vi "QuP Multiplexer Control.vi"(11 "Do full quit? (T)":bool=TRUE) -> ()   [LabVIEW 2020, in "QuPMXdriver.lvlib"]
uses:
  QuPMXdriver.lvlib
  91754cce-ab52-4237-b78a-64c01c446f44.vi
  32ad12f4-2c8c-4504-800a-0d774754ae80.vi
  bf4f7028-8ca7-4759-aadb-7144e2be3c91.vi
  040f1b57-66c1-4072-aa26-6ea72dd8171f.vi
  6aed5eb3-691d-4dc6-b830-00691c629857.vi
  Sequence Editor.vi
  <vilib>/Comparison/Equal/Equal Functor/Equal Functor.lvclass
panel:
  in  "disconnect":bool
  out "dummy for event \"check channels\"":bool
  in  "Set to sequence line:":i32=2 min=1 step=1
  in  "set sq line":bool
  out "Connected\nboards":bool[](array[boolean])
  in  "Get sq from MX":bool
  in  "Load sq to MX":bool
  in  "no sequences get":bool
  out "Number of sequence lines:":i32 min=0 step=1
  in  "sequence editor":bool
  out "Guards ref array":refnum<vi>[][](array[refnum])
  in  "G5C1":bool
  in  "G5C2":bool
  in  "G6C1":bool
  in  "G6C2":bool
  in  "G4C1":bool
  in  "G4C2":bool
  in  "G3C1":bool
  in  "G3C2":bool
  in  "G2C1":bool
  in  "G2C2":bool
  in  "G1C1":bool
  in  "G1C2":bool
  out "No. of connected slave boards:":u32
  out "Slaves ref array":refnum<vi>[][](array[refnum])
  in  "S5C1":bool
  in  "S5C2":bool
  in  "S6C1":bool
  in  "S6C2":bool
  in  "S4C1":bool
  in  "S4C2":bool
  in  "S3C1":bool
  in  "S3C2":bool
  in  "S2C1":bool
  in  "S2C2":bool
  in  "S1C1":bool
  in  "S1C2":bool
  in  "connect":bool
  in  "Get Status":bool
  out "Ready?":bool=TRUE
  out "Enabled":bool=TRUE
  in  "check channels":bool
  in  "delay get":bool
  in  "delay set":bool
  in  "Enable\nDelay (ms)":dbl=2.0 min=0.8
  in  "timer get":bool
  in  "timer set":bool
  in  "Timer (ms)":i32=1000 min=0 step=1
  in  "Trigger polarity":enum32{"Positive", "Negative"}(radio)
  in  "Trigger source":enum32{"Internal", "External"}(radio)
  out "FP":refnum<vi>[](array[refnum])
  in  "Operation":enum32{"Remote", "Local"}(radio)=enum."Local"
  out "ID":string
  in  "reset":bool
  in  "clear":bool
  in  "stop":bool
  in  "start":bool
  in  "resume":bool
  in  "pause":bool
  in  "Close":bool
  out "error":errorcluster
  in  "VISA":refnum<visa-resource-name>
  # "Channels"
  # "Properties"
  # "Slave boards"
  # "1       2      3      4      5      6"
  # "Channel 1"
  # "Channel 2"
  # "1       2      3      4      5      6"
  # "Guards"
  # "Channel 1"
  # "These are buttons,\nclick it!"
  # "Channel 2"
  # "Sequence"
  # "Error"
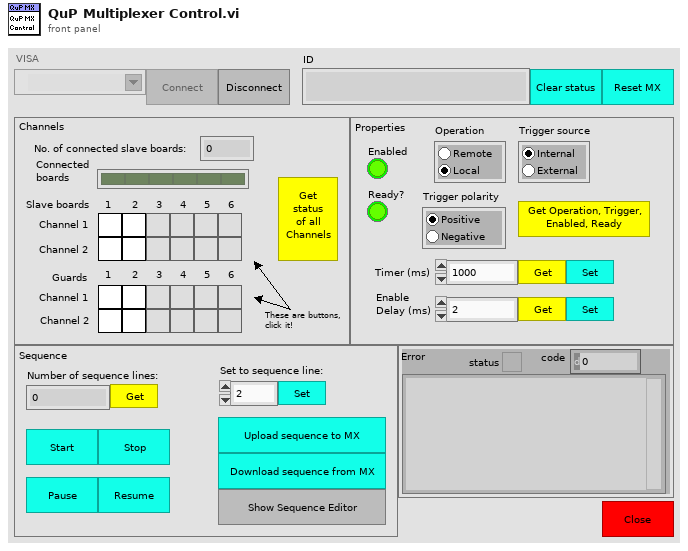
[diagram p1: front panel]
types:
  T1 = enum8{"Enabled", "Disabled", "Disabled and Grayed Out"}
  T2 = enum32{"Invalid", "Standard", "Closed", "Hidden", "Minimized", "Maximized"}
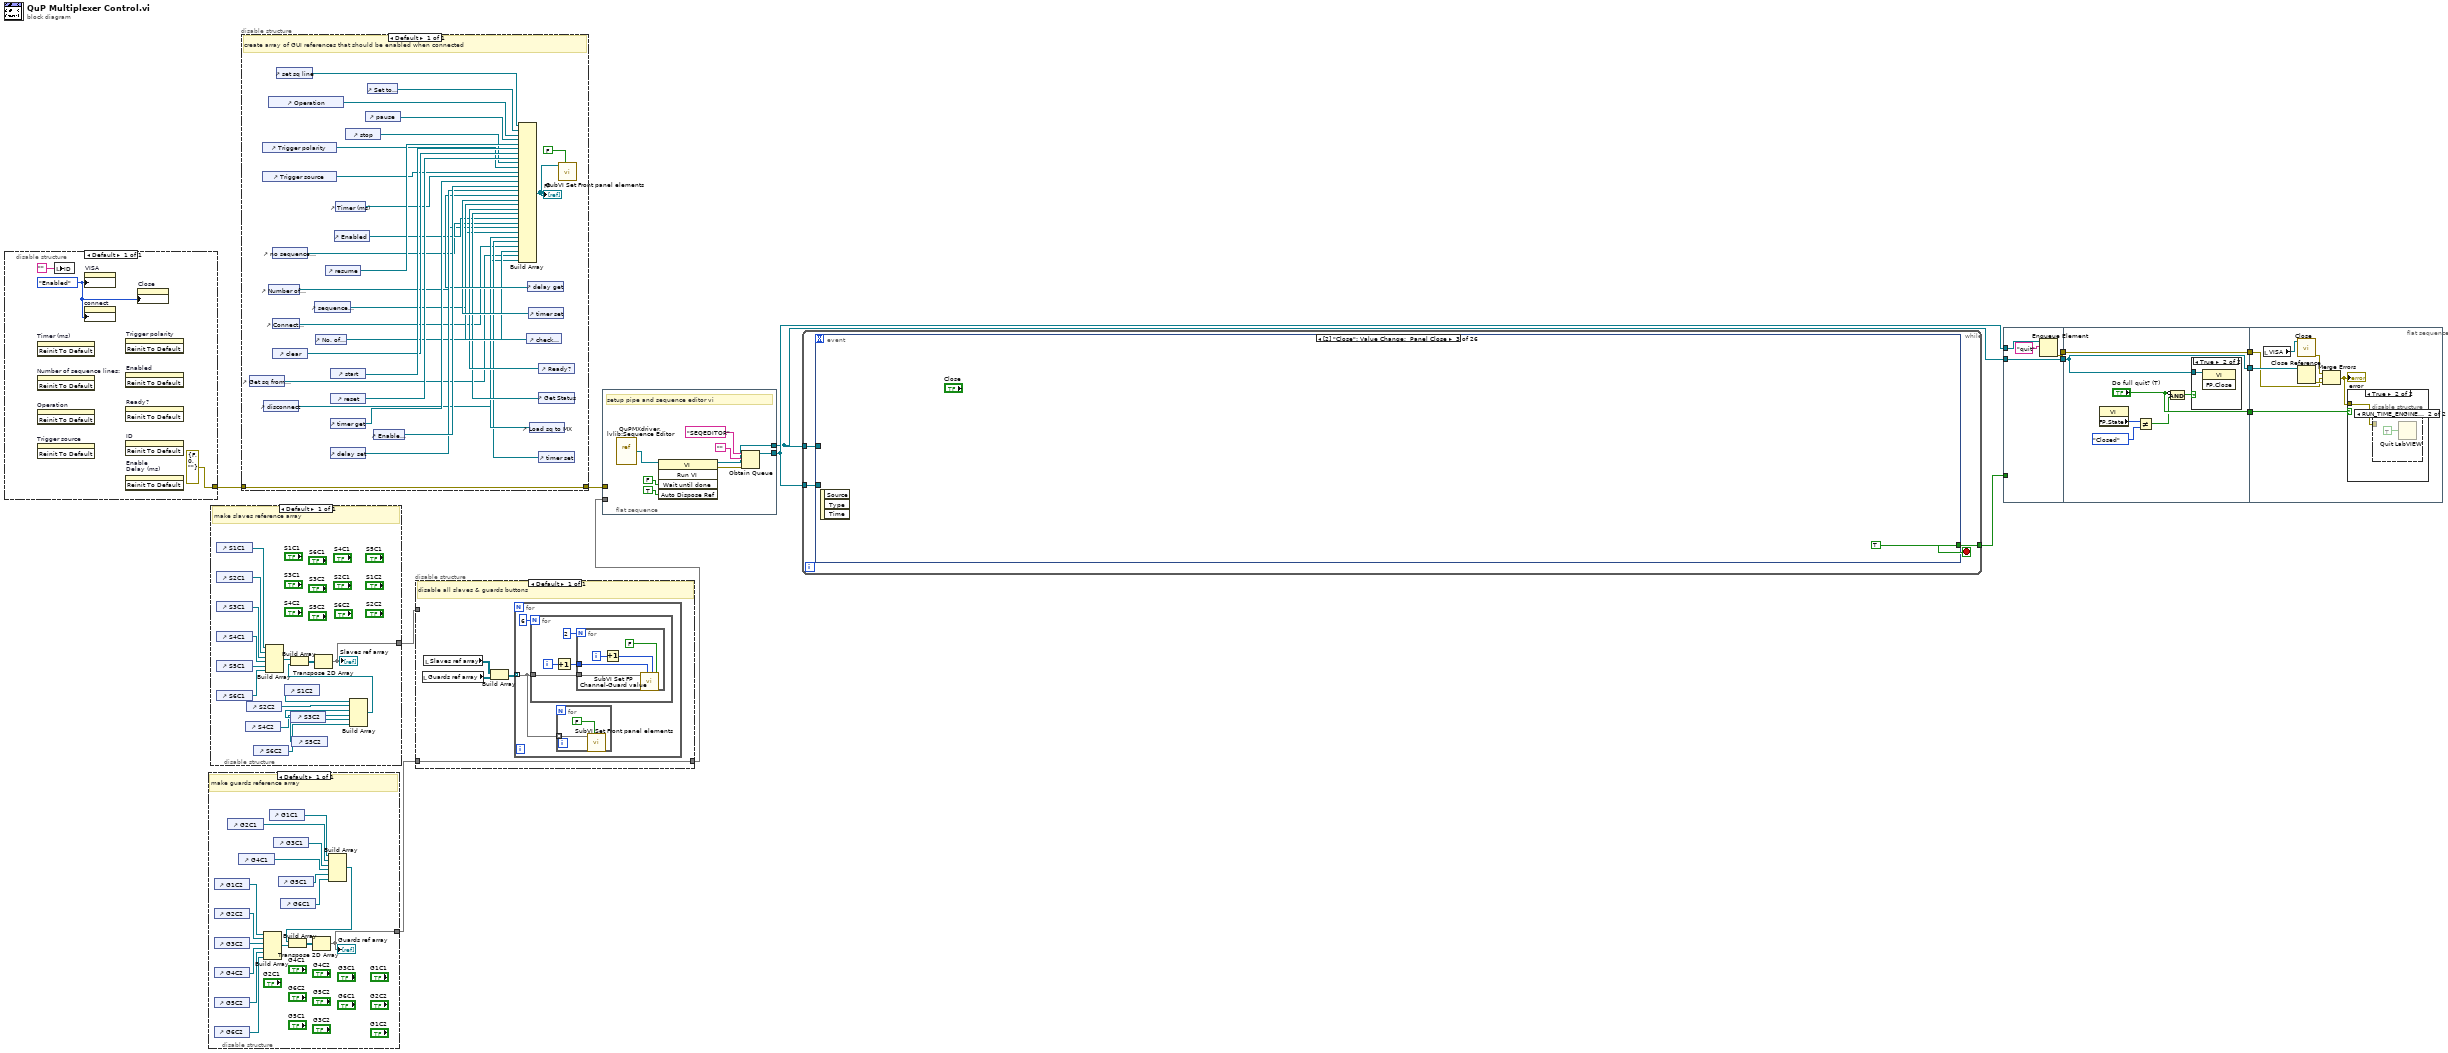
[diagram p0: block diagram]
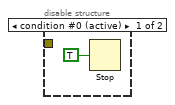
[diagram p4: hidden frame]
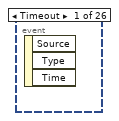
[diagram p5: hidden frame]
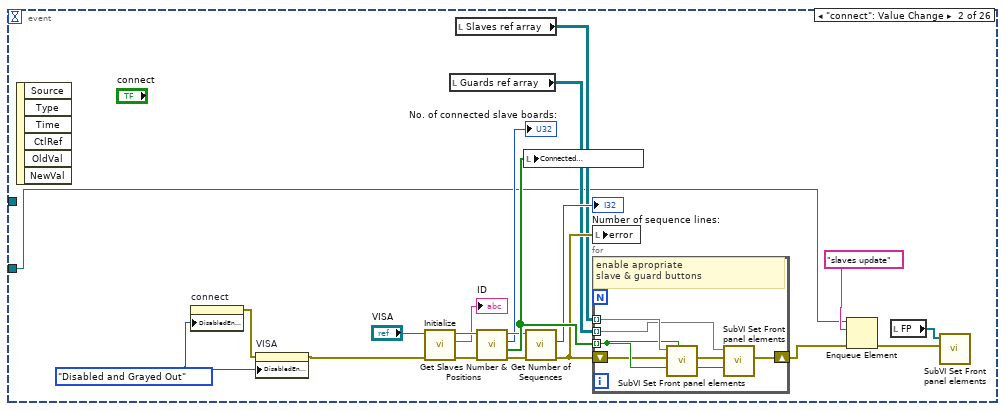
[diagram p6: hidden frame]
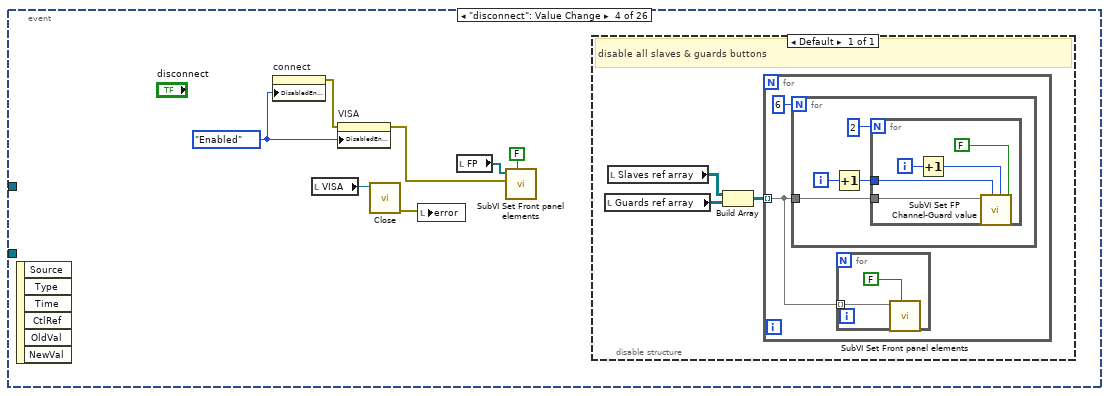
[diagram p7: hidden frame]
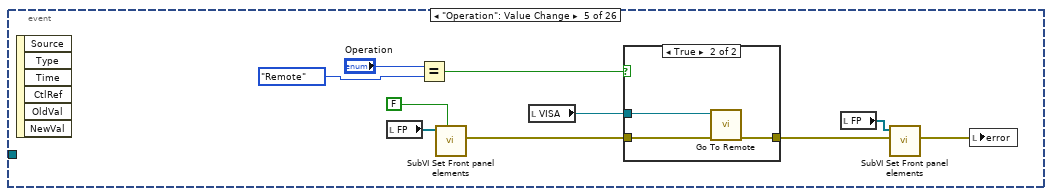
[diagram p8: hidden frame]
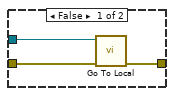
[diagram p9: hidden frame]
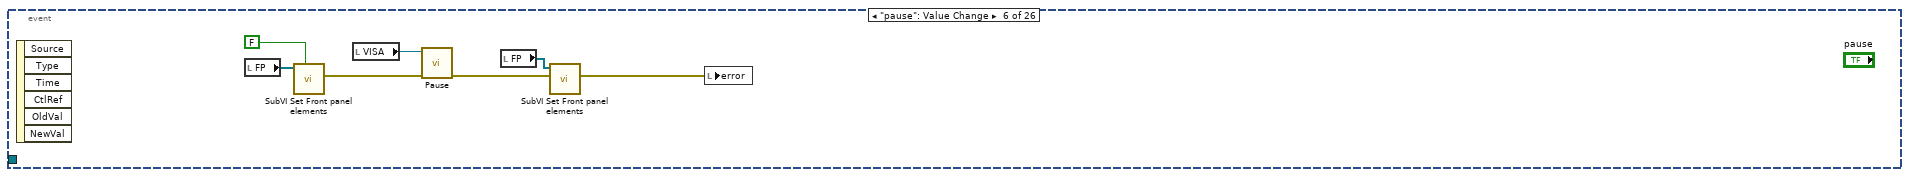
[diagram p10: hidden frame]
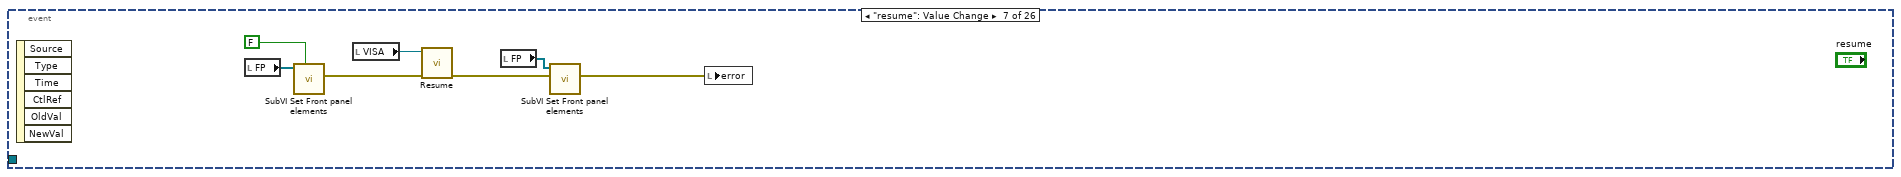
[diagram p11: hidden frame]
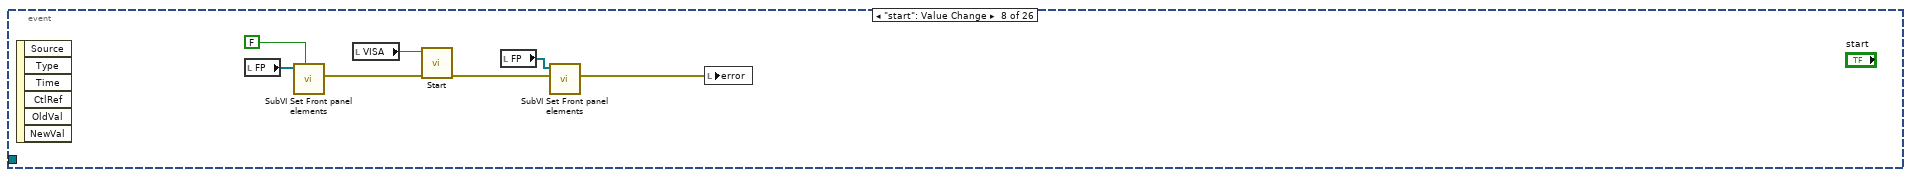
[diagram p12: hidden frame]
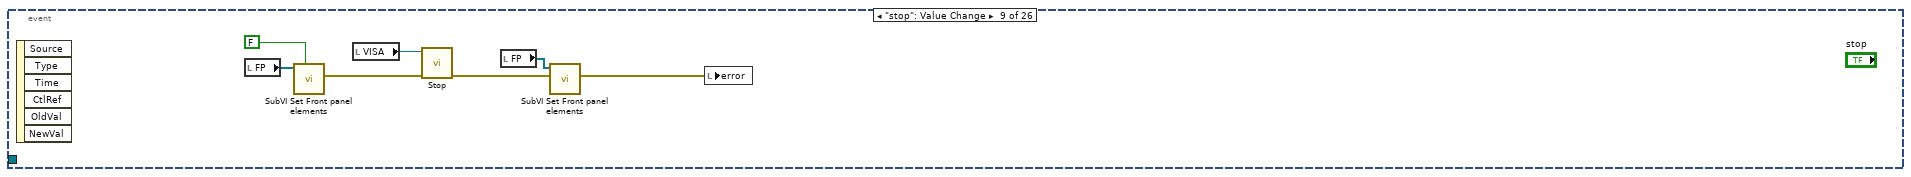
[diagram p13: hidden frame]
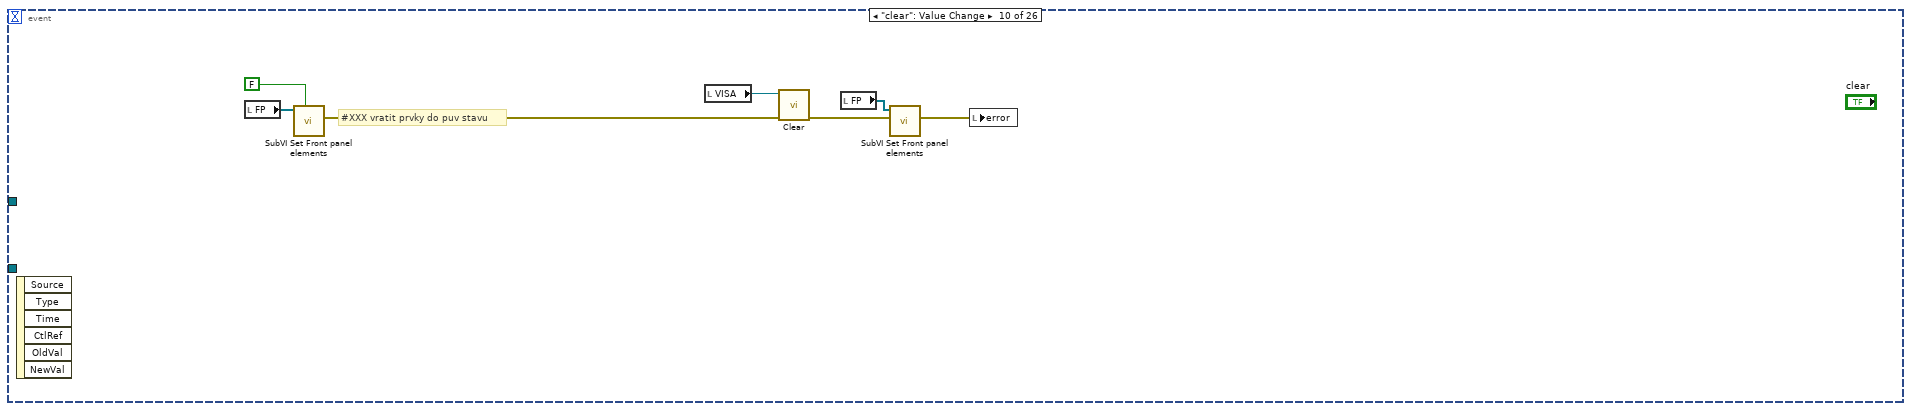
[diagram p14: hidden frame]
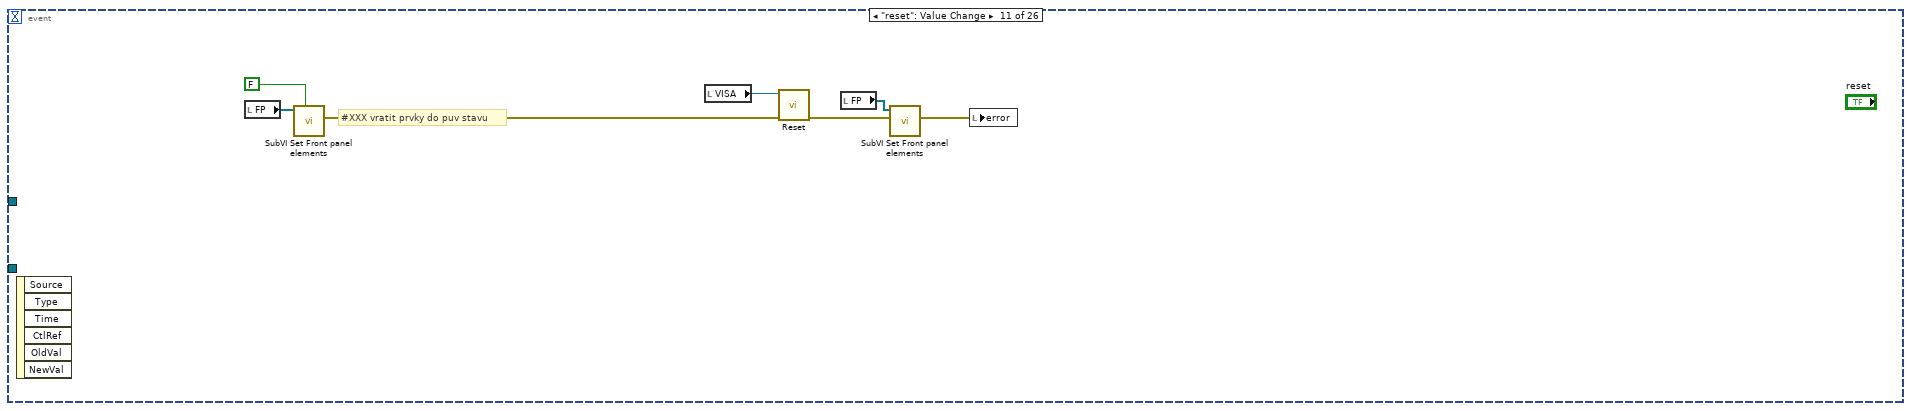
[diagram p15: hidden frame]
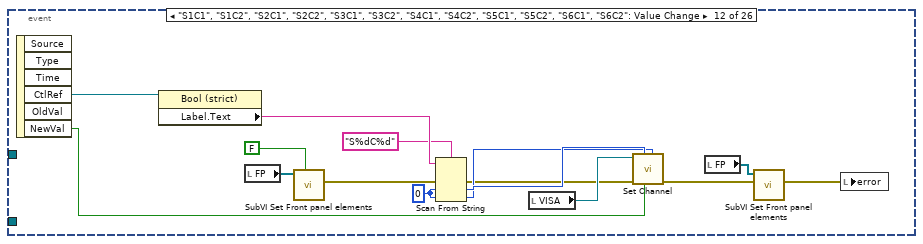
[diagram p16: hidden frame]
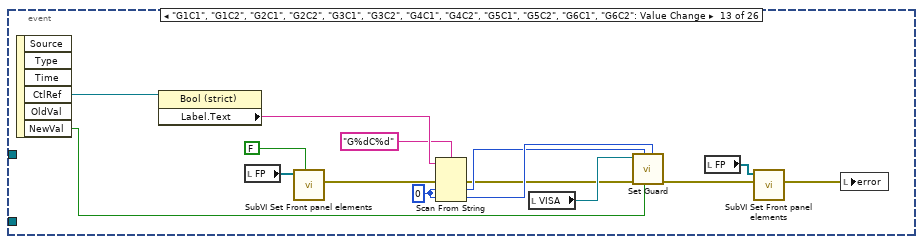
[diagram p17: hidden frame]
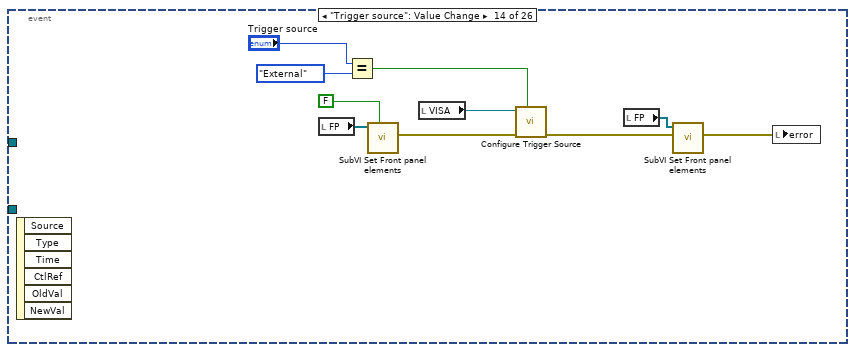
[diagram p18: hidden frame]
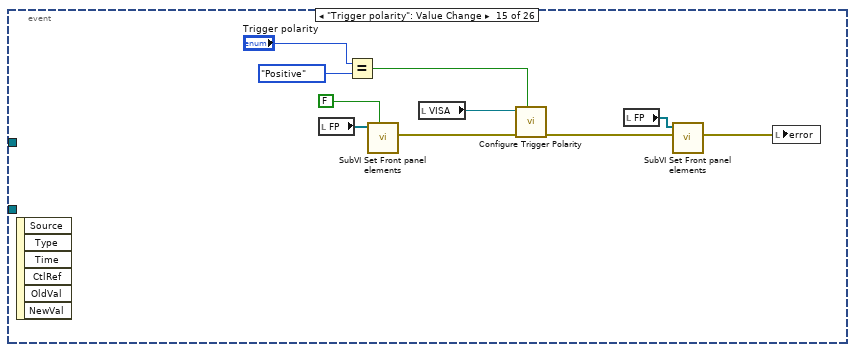
[diagram p19: hidden frame]
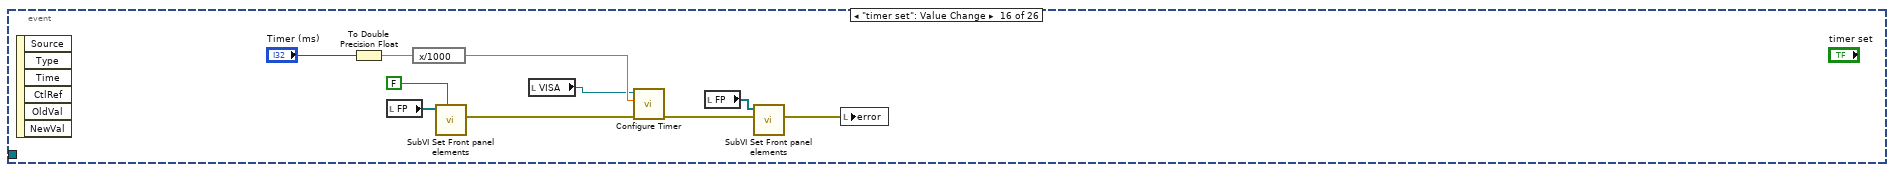
[diagram p20: hidden frame]
diagram:
  n1 = disable-structure shown="Default" {
    disable-tunnel: [errorcluster {"status"=FALSE, "code"=0, "source"=""} ("error in (no error)")] -> w8
    frame Enabled {
      w14 = T1."Enabled" ("Disabled")
      n2 = invoke on="Timer (ms)" class="DigNum (strict)" method="Reinit To Default"() -> ()  [unwired: 3 in, 3 out]
      n3 = invoke on="Number of sequence lines:" class="DigNum (strict)" method="Reinit To Default"() -> ()  [unwired: 3 in, 3 out]
      n4 = invoke on="Operation" class="RadioBtnsControl (strict)" method="Reinit To Default"() -> ()  [unwired: 3 in, 3 out]
      n5 = invoke on="Trigger source" class="RadioBtnsControl (strict)" method="Reinit To Default"() -> ()  [unwired: 3 in, 3 out]
      n6 = local write "ID"("") -> ()
      n7 = property on="VISA" class="VISAName"("DisabledEnum"=w14) -> ()  [unwired: 2 in, 2 out]
      n8 = property on="connect" class="Bool"("DisabledEnum"=w14) -> ()  [unwired: 2 in, 2 out]
      n9 = invoke on="Trigger polarity" class="RadioBtnsControl (strict)" method="Reinit To Default"() -> ()  [unwired: 3 in, 3 out]
      n10 = invoke on="Enabled" class="Bool (strict)" method="Reinit To Default"() -> ()  [unwired: 3 in, 3 out]
      n11 = invoke on="Ready?" class="Bool (strict)" method="Reinit To Default"() -> ()  [unwired: 3 in, 3 out]
      n12 = invoke on="ID" class="Str" method="Reinit To Default"() -> ()  [unwired: 3 in, 3 out]
      n13 = invoke on="Enable\nDelay (ms)" class="DigNum (strict)" method="Reinit To Default"() -> ()  [unwired: 3 in, 3 out]
      n14 = property on="Close" class="Bool"("DisabledEnum"=w14) -> ()  [unwired: 2 in, 2 out]
    }
  }
  n15 = disable-structure shown="Default" {
    disable-tunnel: [w17] -> w11
    frame Enabled {
      # "make guards reference array"
      n16 = control-ref of="G1C2"() -> (w18:refnum<vi>)
      n17 = control-ref of="G2C2"() -> (w19:refnum<vi>)
      n18 = control-ref of="G3C2"() -> (w20:refnum<vi>)
      n19 = control-ref of="G4C2"() -> (w21:refnum<vi>)
      n20 = control-ref of="G5C2"() -> (w22:refnum<vi>)
      n21 = control-ref of="G6C2"() -> (w23:refnum<vi>)
      n22 = control-ref of="G2C1"() -> (w26:refnum<vi>)
      n23 = control-ref of="G4C1"() -> (w28:refnum<vi>)
      n24 = Build Array(w18, w19, w20, w21, w22, w23) -> (w31:refnum<vi>[])
      n25 = control-ref of="G1C1"() -> (w25:refnum<vi>)
      n26 = control-ref of="G3C1"() -> (w27:refnum<vi>)
      n27 = control-ref of="G5C1"() -> (w29:refnum<vi>)
      n28 = control-ref of="G6C1"() -> (w30:refnum<vi>)
      n29 = Build Array(w25, w26, w27, w28, w29, w30) -> (w24:refnum<vi>[])
      n30 = Build Array(w24, w31) -> (w32:refnum<vi>[][])
      n31 = Transpose 2D Array(2D array=w32) -> (transposed array=w17:refnum<vi>[][])
      "Guards ref array" <- w17
    }
  }
  n32 = disable-structure shown="Default" {
    disable-tunnel: [w33] -> w12
    frame Enabled {
      # "make slaves reference array"
      n33 = control-ref of="S1C1"() -> (w48:refnum<vi>)
      n34 = control-ref of="S2C1"() -> (w47:refnum<vi>)
      n35 = control-ref of="S3C1"() -> (w46:refnum<vi>)
      n36 = control-ref of="S4C1"() -> (w45:refnum<vi>)
      n37 = control-ref of="S5C1"() -> (w44:refnum<vi>)
      n38 = control-ref of="S6C1"() -> (w43:refnum<vi>)
      n39 = control-ref of="S4C2"() -> (w39:refnum<vi>)
      n40 = control-ref of="S2C2"() -> (w41:refnum<vi>)
      n41 = control-ref of="S6C2"() -> (w37:refnum<vi>)
      n42 = Build Array(w48, w47, w46, w45, w44, w43) -> (w35:refnum<vi>[])
      n43 = control-ref of="S1C2"() -> (w42:refnum<vi>)
      n44 = control-ref of="S3C2"() -> (w40:refnum<vi>)
      n45 = control-ref of="S5C2"() -> (w38:refnum<vi>)
      n46 = Build Array(w42, w41, w40, w39, w38, w37) -> (w36:refnum<vi>[])
      n47 = Build Array(w35, w36) -> (w34:refnum<vi>[][])
      n48 = Transpose 2D Array(2D array=w34) -> (transposed array=w33:refnum<vi>[][])
      "Slaves ref array" <- w33
    }
  }
  n49 = disable-structure shown="Default" {
    disable-tunnel: [w56] -> w6
    disable-tunnel: w8 -> [w56]
    frame Enabled {
      # "create array of GUI references that should be enabled when connected"
      n50 = control-ref of="Get sq from MX"() -> (w52:refnum<vi>)
      n51 = control-ref of="Trigger polarity"() -> (w72:refnum<vi>)
      n52 = control-ref of="Trigger source"() -> (w71:refnum<vi>)
      n53 = control-ref of="disconnect"() -> (w49:refnum<vi>)
      n54 = control-ref of="Operation"() -> (w81:refnum<vi>)
      n55 = control-ref of="Number of sequence lines:"() -> (w59:refnum<vi>)
      n56 = control-ref of="no sequences get"() -> (w60:refnum<vi>)
      n57 = control-ref of="Connected\nboards"() -> (w54:refnum<vi>)
      n58 = control-ref of="clear"() -> (w77:refnum<vi>)
      n59 = control-ref of="set sq line"() -> (w50:refnum<vi>)
      n60 = control-ref of="sequence editor"() -> (w58:refnum<vi>)
      n61 = control-ref of="No. of connected slave boards:"() -> (w53:refnum<vi>)
      n62 = control-ref of="resume"() -> (w79:refnum<vi>)
      n63 = control-ref of="start"() -> (w78:refnum<vi>)
      n64 = control-ref of="reset"() -> (w76:refnum<vi>)
      n65 = control-ref of="timer get"() -> (w69:refnum<vi>)
      n66 = control-ref of="delay set"() -> (w67:refnum<vi>)
      n67 = control-ref of="Enabled"() -> (w61:refnum<vi>)
      n68 = control-ref of="Timer (ms)"() -> (w70:refnum<vi>)
      n69 = control-ref of="stop"() -> (w73:refnum<vi>)
      n70 = control-ref of="pause"() -> (w80:refnum<vi>)
      n71 = control-ref of="Set to sequence line:"() -> (w51:refnum<vi>)
      n72 = control-ref of="Enable\nDelay (ms)"() -> (w68:refnum<vi>)
      n73 = control-ref of="check channels"() -> (w64:refnum<vi>)
      n74 = control-ref of="delay get"() -> (w66:refnum<vi>)
      n75 = control-ref of="timer set"() -> (w65:refnum<vi>)
      n76 = control-ref of="Load sq to MX"() -> (w57:refnum<vi>)
      n77 = control-ref of="Ready?"() -> (w63:refnum<vi>)
      n78 = control-ref of="Get Status"() -> (w62:refnum<vi>)
      n79 = control-ref of="timer set"() -> (w55:refnum<vi>)
      n80 = Build Array(w50, w51, w81, w80, w79, w78, w77, w76, w73, w72, w71, w70, w69, w68, w67, w66, w65, w64, w63, w62, w61, w60, w59, w58, w57, w55, w54, w53, w52, w49) -> (w75:refnum<vi>[])
      "FP" <- w75
      n81 = call "SubVI Set Front panel elements.vi"("Enable elements (T)"=FALSE ("Enable elements"), "Array"=w75) -> ()  [unwired: 9 in, 1 out]
    }
  }
  n82 = disable-structure shown="Default" {
    disable-tunnel: w12 -> [_]
    disable-tunnel: w11 -> [w82]
    disable-tunnel: [w82] -> w7
    frame Enabled {
      # "disable all slaves & guards buttons"
      n83 = local read "Guards ref array"() -> (w83:refnum<vi>[][])
      n84 = local read "Slaves ref array"() -> (w85:refnum<vi>[][])
      n85 = Build Array(w85, w83) -> (w84:refnum<vi>[][][])
      n86 = for {
        tunnel: w84 -> [w86] mode=indexing
        n87 = for {
          N: 6 -> [_]
          tunnel: w86 -> [w91]
          i -> [w89]
          n88 = Increment(x=w89) -> (x+1=w88:i32)
          n89 = for {
            N: 2 -> [_]
            tunnel: w91 -> [w96]
            tunnel: w88 -> [w94]
            i -> [w93]
            n90 = Increment(x=w93) -> (x+1=w92:i32)
            n91 = call "SubVI Set FP Channel-Guard value.vi"("Value"=FALSE, "Ch ID"=w92, "Slave ID"=w94, "Slaves ref array"=w96) -> ()  [unwired: 7 in, 1 out]
          }
        }
        n92 = for {
          tunnel: w86 -> [w98] mode=indexing
          n93 = call "SubVI Set Front panel elements.vi"("Enable elements (T)"=FALSE, "Array"=w98) -> ()  [unwired: 9 in, 1 out]
        }
      }
    }
  }
  n94 = flat-sequence {
    tunnel: [w99] -> w10
    tunnel: [w101] -> w9
    tunnel: w7 -> [_]
    tunnel: w6 -> [_]
    frame #0 {
      # "setup pipe and sequence editor vi"
      n95 = vi-ref "QuPMXdriver.lvlib:Sequence Editor.vi"() -> (w106:refnum<vi>)
      n96 = invoke class="VI" method="Run VI"(reference=w106, "Wait until done"=FALSE ("Wait Until Done"), "Auto Dispose Ref"=TRUE ("Wait Until Done")) -> (reference out=w101:refnum<vi>, error out=w102:errorcluster)  [unwired: 2 in, 3 out]
      n97 = Obtain Queue(name (unnamed)="SEQEDITOR", element data type="", error in (no error)=w102) -> (queue out=w99:refnum<queue>)  [unwired: 2 in, 2 out]
    }
  }
  n98 = while {
    tunnel: [w109] -> w13
    tunnel: w10 -> [w108]
    tunnel: w9 -> [w107]
    stop <- w109 stop-if-true
    n99 = event shown="[2] \"Close\": Value Change;  Panel Close" {
      selector: _ -> [_ _ _ _ _ _ _ _ _ _ _ _ _ _ _ _ _ _ _ _ _ _ _ _ _ _]
      dyn-events: _ -> [_ _ _ _ _ _ _ _ _ _ _ _ _ _ _ _ _ _ _ _ _ _ _ _ _ _]
      timeout: _ -> [_ _ _ _ _ _ _ _ _ _ _ _ _ _ _ _ _ _ _ _ _ _ _ _ _ _]
      tunnel: [_ _ TRUE ("Stop") _ _ _ _ _ _ _ _ _ _ _ _ _ _ _ _ _ _ _ _ _ _ _] -> w109
      tunnel: w108 -> [_ w110 _ _ _ _ _ _ _ _ _ _ _ _ _ _ _ _ _ w307 _ _ w371 _ _ w448]
      tunnel: w107 -> [_ _ _ _ _ _ _ _ _ _ _ _ _ _ _ _ _ _ _ _ _ _ _ w376 w424 w451]
      event Timeout {
        n100 = event-data() -> ()  [unwired: 1 in, 3 out]
      }
      event "connect": Value Change {
        w116 = T1."Disabled and Grayed Out" ("Disabled")
        n101 = event-data() -> ()  [unwired: 1 in, 6 out]
        n102 = property on="connect" class="Bool"("DisabledEnum"=w116) -> (error out=w117:errorcluster)  [unwired: 2 in, 1 out]
        n103 = property on="VISA" class="VISAName"(error in=w117, "DisabledEnum"=w116) -> (error out=w115:errorcluster)  [unwired: 1 in, 1 out]
        n104 = call "Initialize.vi"("error in (no error)"=w115, "VISA resource name"="VISA") -> ("error out"=w119:errorcluster, "ID"=→"ID":string, "VISA resource name out"=w120:refnum<visa-resource-name>)  [unwired: 7 in]
        n105 = local read "Guards ref array"() -> (w123:refnum<vi>[][])
        n106 = local read "Slaves ref array"() -> (w122:refnum<vi>[][])
        n107 = call "Get Slaves Number & Positions.vi"("error in (no error)"=w119, "VISA resource name"=w120) -> ("error out"=w124:errorcluster, "Connected Slaves"=w129:bool[], "No. of Slaves"=→"No. of connected slave boards:":u32, "VISA resource name out"=w126:refnum<visa-resource-name>)  [unwired: 6 in]
        n108 = local write "Connected\nboards"(w129) -> ()
        n109 = call "Get Number of Sequences.vi"("error in (no error)"=w124, "VISA resource name"=w126) -> ("error out"=w125:errorcluster, "Number of sequences"=→"Number of sequence lines:":i32)  [unwired: 7 in, 1 out]
        n110 = local write "error"(w125) -> ()
        n111 = for {
          tunnel: w122 -> [w135] mode=indexing
          tunnel: w129 -> [w133] mode=indexing
          tunnel: w123 -> [w134] mode=indexing
          shift-right: [w131] -> w111
          shift-left: w125 -> [w130]
          # "enable apropriate\nslave & guard buttons"
          n112 = call "SubVI Set Front panel elements.vi"("Enable elements (T)"=w133, "error in (passthrough)"=w130, "Array"=w135) -> ("error out"=w132:errorcluster)  [unwired: 8 in]
          n113 = call "SubVI Set Front panel elements.vi"("Enable elements (T)"=w133, "error in (passthrough)"=w132, "Array"=w134) -> ("error out"=w131:errorcluster)  [unwired: 8 in]
        }
        n114 = Enqueue Element(queue=w110, element="slaves update", error in (no error)=w111) -> (error out=w114:errorcluster)  [unwired: 1 in, 2 out]
        n115 = local read "FP"() -> (w113:refnum<vi>[])
        n116 = call "SubVI Set Front panel elements.vi"("error in (passthrough)"=w114, "Array"=w113) -> ()  [unwired: 9 in, 1 out]
      }
      event "Close": Value Change; Panel Close {
        n117 = event-data() -> ()  [unwired: 1 in, 3 out]
      }
      event "disconnect": Value Change {
        w141 = T1."Enabled" ("Disabled")
        n118 = event-data() -> ()  [unwired: 1 in, 6 out]
        n119 = property on="connect" class="Bool"("DisabledEnum"=w141) -> (error out=w142:errorcluster)  [unwired: 2 in, 1 out]
        n120 = local read "VISA"() -> (w143:refnum<visa-resource-name>)
        n121 = property on="VISA" class="VISAName"(error in=w142, "DisabledEnum"=w141) -> (error out=w138:errorcluster)  [unwired: 1 in, 1 out]
        n122 = call "Close.vi"("VISA resource name"=w143) -> ("error out"=w140:errorcluster)  [unwired: 10 in]
        n123 = local write "error"(w140) -> ()
        n124 = local read "FP"() -> (w139:refnum<vi>[])
        n125 = call "SubVI Set Front panel elements.vi"("Enable elements (T)"=FALSE, "error in (passthrough)"=w138, "Array"=w139) -> ()  [unwired: 8 in, 1 out]
        n126 = disable-structure shown="Default" {
          frame Enabled {
            # "disable all slaves & guards buttons"
            n127 = local read "Guards ref array"() -> (w144:refnum<vi>[][])
            n128 = local read "Slaves ref array"() -> (w146:refnum<vi>[][])
            n129 = Build Array(w146, w144) -> (w145:refnum<vi>[][][])
            n130 = for {
              tunnel: w145 -> [w147] mode=indexing
              n131 = for {
                N: 6 -> [_]
                tunnel: w147 -> [w152]
                i -> [w150]
                n132 = Increment(x=w150) -> (x+1=w149:i32)
                n133 = for {
                  N: 2 -> [_]
                  tunnel: w152 -> [w157]
                  tunnel: w149 -> [w155]
                  i -> [w154]
                  n134 = Increment(x=w154) -> (x+1=w153:i32)
                  n135 = call "SubVI Set FP Channel-Guard value.vi"("Value"=FALSE, "Ch ID"=w153, "Slave ID"=w155, "Slaves ref array"=w157) -> ()  [unwired: 7 in, 1 out]
                }
              }
              n136 = for {
                tunnel: w147 -> [w159] mode=indexing
                n137 = call "SubVI Set Front panel elements.vi"("Enable elements (T)"=FALSE, "Array"=w159) -> ()  [unwired: 9 in, 1 out]
              }
            }
          }
        }
      }
      event "Operation": Value Change {
        n138 = event-data() -> ()  [unwired: 1 in, 6 out]
        n139 = local read "FP"() -> (w165:refnum<vi>[])
        n140 = Equal?(x="Operation", y=enum32{"Remote", "Local"}."Remote") -> (x = y?=w166:bool)
        n141 = call "SubVI Set Front panel elements.vi"("Enable elements (T)"=FALSE, "Array"=w165) -> ("error out"=w163:errorcluster)  [unwired: 9 in]
        n142 = local read "VISA"() -> (w169:refnum<visa-resource-name>)
        n143 = case shown="True" w166 {
          tunnel: [w172 w175] -> w162
          tunnel: w169 -> [w171 w174]
          tunnel: w163 -> [w170 w173]
          frame False {
            n144 = call "Go To Local.vi"("error in (no error)"=w170, "VISA resource name"=w171) -> ("error out"=w172:errorcluster)  [unwired: 8 in, 1 out]
          }
          frame True {
            n145 = call "Go To Remote.vi"("error in (no error)"=w173, "VISA resource name"=w174) -> ("error out"=w175:errorcluster)  [unwired: 8 in, 1 out]
          }
        }
        n146 = local read "FP"() -> (w160:refnum<vi>[])
        n147 = call "SubVI Set Front panel elements.vi"("error in (passthrough)"=w162, "Array"=w160) -> ("error out"=w161:errorcluster)  [unwired: 9 in]
        n148 = local write "error"(w161) -> ()
      }
      event "pause": Value Change {
        n149 = event-data() -> ()  [unwired: 1 in, 6 out]
        n150 = local read "FP"() -> (w181:refnum<vi>[])
        n151 = call "SubVI Set Front panel elements.vi"("Enable elements (T)"=FALSE, "Array"=w181) -> ("error out"=w178:errorcluster)  [unwired: 9 in]
        n152 = local read "VISA"() -> (w182:refnum<visa-resource-name>)
        n153 = call "Pause.vi"("error in (no error)"=w178, "VISA resource name"=w182) -> ("error out"=w177:errorcluster)  [unwired: 8 in, 1 out]
        n154 = local read "FP"() -> (w179:refnum<vi>[])
        n155 = call "SubVI Set Front panel elements.vi"("error in (passthrough)"=w177, "Array"=w179) -> ("error out"=w176:errorcluster)  [unwired: 9 in]
        n156 = local write "error"(w176) -> ()
      }
      event "resume": Value Change {
        n157 = event-data() -> ()  [unwired: 1 in, 6 out]
        n158 = local read "FP"() -> (w187:refnum<vi>[])
        n159 = call "SubVI Set Front panel elements.vi"("Enable elements (T)"=FALSE, "Array"=w187) -> ("error out"=w185:errorcluster)  [unwired: 9 in]
        n160 = local read "VISA"() -> (w189:refnum<visa-resource-name>)
        n161 = call "Resume.vi"("error in (no error)"=w185, "VISA resource name"=w189) -> ("error out"=w184:errorcluster)  [unwired: 8 in, 1 out]
        n162 = local read "FP"() -> (w188:refnum<vi>[])
        n163 = call "SubVI Set Front panel elements.vi"("error in (passthrough)"=w184, "Array"=w188) -> ("error out"=w183:errorcluster)  [unwired: 9 in]
        n164 = local write "error"(w183) -> ()
      }
      event "start": Value Change {
        n165 = event-data() -> ()  [unwired: 1 in, 6 out]
        n166 = local read "FP"() -> (w194:refnum<vi>[])
        n167 = call "SubVI Set Front panel elements.vi"("Enable elements (T)"=FALSE, "Array"=w194) -> ("error out"=w192:errorcluster)  [unwired: 9 in]
        n168 = local read "VISA"() -> (w196:refnum<visa-resource-name>)
        n169 = call "Start.vi"("error in (no error)"=w192, "VISA resource name"=w196) -> ("error out"=w191:errorcluster)  [unwired: 8 in, 1 out]
        n170 = local read "FP"() -> (w195:refnum<vi>[])
        n171 = call "SubVI Set Front panel elements.vi"("error in (passthrough)"=w191, "Array"=w195) -> ("error out"=w190:errorcluster)  [unwired: 9 in]
        n172 = local write "error"(w190) -> ()
      }
      event "stop": Value Change {
        n173 = event-data() -> ()  [unwired: 1 in, 6 out]
        n174 = local read "FP"() -> (w201:refnum<vi>[])
        n175 = call "SubVI Set Front panel elements.vi"("Enable elements (T)"=FALSE, "Array"=w201) -> ("error out"=w199:errorcluster)  [unwired: 9 in]
        n176 = local read "VISA"() -> (w203:refnum<visa-resource-name>)
        n177 = call "Stop.vi"("error in (no error)"=w199, "VISA resource name"=w203) -> ("error out"=w198:errorcluster)  [unwired: 8 in, 1 out]
        n178 = local read "FP"() -> (w202:refnum<vi>[])
        n179 = call "SubVI Set Front panel elements.vi"("error in (passthrough)"=w198, "Array"=w202) -> ("error out"=w197:errorcluster)  [unwired: 9 in]
        n180 = local write "error"(w197) -> ()
      }
      event "clear": Value Change {
        # "#XXX vratit prvky do puv stavu"
        n181 = event-data() -> ()  [unwired: 1 in, 6 out]
        n182 = local read "FP"() -> (w208:refnum<vi>[])
        n183 = call "SubVI Set Front panel elements.vi"("Enable elements (T)"=FALSE, "Array"=w208) -> ("error out"=w206:errorcluster)  [unwired: 9 in]
        n184 = local read "VISA"() -> (w210:refnum<visa-resource-name>)
        n185 = call "Clear.vi"("error in (no error)"=w206, "VISA resource name"=w210) -> ("error out"=w205:errorcluster)  [unwired: 8 in, 1 out]
        n186 = local read "FP"() -> (w209:refnum<vi>[])
        n187 = call "SubVI Set Front panel elements.vi"("error in (passthrough)"=w205, "Array"=w209) -> ("error out"=w204:errorcluster)  [unwired: 9 in]
        n188 = local write "error"(w204) -> ()
      }
      event "reset": Value Change {
        # "#XXX vratit prvky do puv stavu"
        n189 = event-data() -> ()  [unwired: 1 in, 6 out]
        n190 = local read "FP"() -> (w215:refnum<vi>[])
        n191 = call "SubVI Set Front panel elements.vi"("Enable elements (T)"=FALSE, "Array"=w215) -> ("error out"=w213:errorcluster)  [unwired: 9 in]
        n192 = local read "VISA"() -> (w217:refnum<visa-resource-name>)
        n193 = call "Reset.vi"("error in (no error)"=w213, "VISA resource name"=w217) -> ("error out"=w212:errorcluster)  [unwired: 8 in, 1 out]
        n194 = local read "FP"() -> (w216:refnum<vi>[])
        n195 = call "SubVI Set Front panel elements.vi"("error in (passthrough)"=w212, "Array"=w216) -> ("error out"=w211:errorcluster)  [unwired: 9 in]
        n196 = local write "error"(w211) -> ()
      }
      event "S1C1", "S1C2", "S2C1", "S2C2", "S3C1", "S3C2", "S4C1", "S4C2", "S5C1", "S5C2", "S6C1", "S6C2": Value Change {
        w218 = 0 ("default value 1")
        n197 = event-data() -> ("CtlRef"=w232:refnum<vi>, "NewVal"=w226:bool)  [unwired: 1 in, 4 out]
        n198 = property class="Bool (strict)"(reference=w232) -> ("Label.Text"=w231:string)  [unwired: 1 in, 2 out]
        n199 = local read "FP"() -> (w221:refnum<vi>[])
        n200 = call "SubVI Set Front panel elements.vi"("Enable elements (T)"=FALSE, "Array"=w221) -> ("error out"=w219:errorcluster)  [unwired: 9 in]
        n201 = Scan From String(format string="S%dC%d", input string=w231, error in=w219, default 1=w218, default 2=w218) -> (error out=w225:errorcluster, output 1=w229:i32, output 2=w228:i32)  [unwired: 1 in, 2 out]
        n202 = local read "VISA"() -> (w227:refnum<visa-resource-name>)
        n203 = call "Set Channel.vi"("Channel"=w228, "Channel Status"=w226, "Slave"=w229, "error in (no error)"=w225, "VISA resource name"=w227) -> ("error out"=w223:errorcluster)  [unwired: 5 in, 1 out]
        n204 = local read "FP"() -> (w224:refnum<vi>[])
        n205 = call "SubVI Set Front panel elements.vi"("error in (passthrough)"=w223, "Array"=w224) -> ("error out"=w222:errorcluster)  [unwired: 9 in]
        n206 = local write "error"(w222) -> ()
      }
      event "G1C1", "G1C2", "G2C1", "G2C2", "G3C1", "G3C2", "G4C1", "G4C2", "G5C1", "G5C2", "G6C1", "G6C2": Value Change {
        w239 = 0 ("default value 1")
        n207 = event-data() -> ("CtlRef"=w245:refnum<vi>, "NewVal"=w241:bool)  [unwired: 1 in, 4 out]
        n208 = property class="Bool (strict)"(reference=w245) -> ("Label.Text"=w247:string)  [unwired: 1 in, 2 out]
        n209 = local read "FP"() -> (w238:refnum<vi>[])
        n210 = call "SubVI Set Front panel elements.vi"("Enable elements (T)"=FALSE, "Array"=w238) -> ("error out"=w236:errorcluster)  [unwired: 9 in]
        n211 = Scan From String(format string="G%dC%d", input string=w247, error in=w236, default 1=w239, default 2=w239) -> (error out=w240:errorcluster, output 1=w243:i32, output 2=w244:i32)  [unwired: 1 in, 2 out]
        n212 = local read "VISA"() -> (w242:refnum<visa-resource-name>)
        n213 = call "Set Guard.vi"("Channel"=w244, "Channel Guard Status"=w241, "Slave"=w243, "error in (no error)"=w240, "VISA resource name"=w242) -> ("error out"=w234:errorcluster)  [unwired: 5 in, 1 out]
        n214 = local read "FP"() -> (w235:refnum<vi>[])
        n215 = call "SubVI Set Front panel elements.vi"("error in (passthrough)"=w234, "Array"=w235) -> ("error out"=w233:errorcluster)  [unwired: 9 in]
        n216 = local write "error"(w233) -> ()
      }
      event "Trigger source": Value Change {
        n217 = event-data() -> ()  [unwired: 1 in, 6 out]
        n218 = local read "FP"() -> (w255:refnum<vi>[])
        n219 = Equal?(x="Trigger source", y=enum32{"Internal", "External"}."External") -> (x = y?=w249:bool)
        n220 = call "SubVI Set Front panel elements.vi"("Enable elements (T)"=FALSE, "Array"=w255) -> ("error out"=w251:errorcluster)  [unwired: 9 in]
        n221 = local read "VISA"() -> (w253:refnum<visa-resource-name>)
        n222 = call "Configure Trigger Source.vi"("Trigger External (T)"=w249, "error in (no error)"=w251, "VISA resource name"=w253) -> ("error out"=w252:errorcluster)  [unwired: 7 in, 1 out]
        n223 = local read "FP"() -> (w256:refnum<vi>[])
        n224 = call "SubVI Set Front panel elements.vi"("error in (passthrough)"=w252, "Array"=w256) -> ("error out"=w257:errorcluster)  [unwired: 9 in]
        n225 = local write "error"(w257) -> ()
      }
      event "Trigger polarity": Value Change {
        n226 = event-data() -> ()  [unwired: 1 in, 6 out]
        n227 = local read "FP"() -> (w265:refnum<vi>[])
        n228 = Equal?(x="Trigger polarity", y=enum32{"Positive", "Negative"}."Positive") -> (x = y?=w259:bool)
        n229 = call "SubVI Set Front panel elements.vi"("Enable elements (T)"=FALSE, "Array"=w265) -> ("error out"=w263:errorcluster)  [unwired: 9 in]
        n230 = local read "VISA"() -> (w258:refnum<visa-resource-name>)
        n231 = call "Configure Trigger Polarity.vi"("Trigger Polarity Positive (T)"=w259, "error in (no error)"=w263, "VISA resource name"=w258) -> ("error out"=w262:errorcluster)  [unwired: 7 in, 1 out]
        n232 = local read "FP"() -> (w266:refnum<vi>[])
        n233 = call "SubVI Set Front panel elements.vi"("error in (passthrough)"=w262, "Array"=w266) -> ("error out"=w267:errorcluster)  [unwired: 9 in]
        n234 = local write "error"(w267) -> ()
      }
      event "timer set": Value Change {
        n235 = event-data() -> ()  [unwired: 1 in, 6 out]
        n236 = To Double Precision Float(number="Timer (ms)") -> (double precision float=w272:dbl)
        n237 = local read "FP"() -> (w275:refnum<vi>[])
        n238 = expression code="x/1000"(w272) -> (w271:dbl)
        n239 = call "SubVI Set Front panel elements.vi"("Enable elements (T)"=FALSE, "Array"=w275) -> ("error out"=w269:errorcluster)  [unwired: 9 in]
        n240 = local read "VISA"() -> (w270:refnum<visa-resource-name>)
        n241 = call "Configure Timer.vi"("error in (no error)"=w269, "Internal timer (2 s)"=w271, "VISA resource name"=w270) -> ("error out"=w268:errorcluster)  [unwired: 7 in, 1 out]
        n242 = local read "FP"() -> (w276:refnum<vi>[])
        n243 = call "SubVI Set Front panel elements.vi"("error in (passthrough)"=w268, "Array"=w276) -> ("error out"=w277:errorcluster)  [unwired: 9 in]
        n244 = local write "error"(w277) -> ()
      }
      event "timer get": Value Change {
        n245 = event-data() -> ()  [unwired: 1 in, 6 out]
        n246 = local read "FP"() -> (w284:refnum<vi>[])
        n247 = call "SubVI Set Front panel elements.vi"("Enable elements (T)"=FALSE, "Array"=w284) -> ("error out"=w282:errorcluster)  [unwired: 9 in]
        n248 = local read "VISA"() -> (w280:refnum<visa-resource-name>)
        n249 = call "Get Timer.vi"("error in (no error)"=w282, "VISA resource name"=w280) -> ("error out"=w281:errorcluster, "Internal Timer value (s)"=w279:dbl)  [unwired: 7 in, 1 out]
        n250 = expression code="int(x*1000)"(w279) -> (w278:dbl)
        n251 = local read "FP"() -> (w285:refnum<vi>[])
        n252 = call "SubVI Set Front panel elements.vi"("error in (passthrough)"=w281, "Array"=w285) -> ("error out"=w286:errorcluster)  [unwired: 9 in]
        n253 = local write "Timer (ms)"(w278) -> ()
        n254 = local write "error"(w286) -> ()
      }
      event "delay set": Value Change {
        n255 = event-data() -> ()  [unwired: 1 in, 6 out]
        n256 = local read "FP"() -> (w293:refnum<vi>[])
        n257 = expression code="x/1000"("Enable\nDelay (ms)") -> (w288:dbl)
        n258 = call "SubVI Set Front panel elements.vi"("Enable elements (T)"=FALSE, "Array"=w293) -> ("error out"=w290:errorcluster)  [unwired: 9 in]
        n259 = local read "VISA"() -> (w291:refnum<visa-resource-name>)
        n260 = call "Configure Delay.vi"("error in (no error)"=w290, "Delay (s)"=w288, "VISA resource name"=w291) -> ("error out"=w289:errorcluster)  [unwired: 7 in, 1 out]
        n261 = local read "FP"() -> (w294:refnum<vi>[])
        n262 = call "SubVI Set Front panel elements.vi"("error in (passthrough)"=w289, "Array"=w294) -> ("error out"=w295:errorcluster)  [unwired: 9 in]
        n263 = local write "error"(w295) -> ()
      }
      event "delay get": Value Change {
        n264 = event-data() -> ()  [unwired: 1 in, 6 out]
        n265 = local read "FP"() -> (w302:refnum<vi>[])
        n266 = call "SubVI Set Front panel elements.vi"("Enable elements (T)"=FALSE, "Array"=w302) -> ("error out"=w300:errorcluster)  [unwired: 9 in]
        n267 = local read "VISA"() -> (w298:refnum<visa-resource-name>)
        n268 = call "Get Delay.vi"("error in (no error)"=w300, "VISA resource name"=w298) -> ("error out"=w299:errorcluster, "Delay (s)"=w297:dbl)  [unwired: 7 in, 1 out]
        n269 = expression code="int(x*1000)"(w297) -> (w296:dbl)
        n270 = local read "FP"() -> (w303:refnum<vi>[])
        n271 = call "SubVI Set Front panel elements.vi"("error in (passthrough)"=w299, "Array"=w303) -> ("error out"=w304:errorcluster)  [unwired: 9 in]
        n272 = local write "Enable\nDelay (ms)"(w296) -> ()
        n273 = local write "error"(w304) -> ()
      }
      event "check channels", "dummy for event \"check channels\"": Value Change {
        # "this is only to get possibility\nto start this event case\neven if button \"check channels\"\nis latching"
        n274 = event-data() -> ()  [unwired: 1 in, 6 out]
        n275 = local read "FP"() -> (w319:refnum<vi>[])
        n276 = call "SubVI Set Front panel elements.vi"("Enable elements (T)"=FALSE, "Array"=w319) -> ("error out"=w312:errorcluster)  [unwired: 9 in]
        n277 = local read "VISA"() -> (w313:refnum<visa-resource-name>)
        n278 = local read "Guards ref array"() -> (w309:refnum<vi>[][])
        n279 = local read "Slaves ref array"() -> (w315:refnum<vi>[][])
        n280 = call "Get Slaves Number & Positions.vi"("error in (no error)"=w312, "VISA resource name"=w313) -> ("error out"=w310:errorcluster, "Connected Slaves"=w314:bool[], "No. of Slaves"=w316:u32)  [unwired: 6 in, 1 out]
        "Connected\nboards" <- w314
        n281 = local write "No. of connected slave boards:"(w316) -> ()
        n282 = for {
          tunnel: w315 -> [w327] mode=indexing
          tunnel: w314 -> [w323] mode=indexing
          shift-right: [w324] -> w311
          shift-left: w310 -> [w326]
          tunnel: w309 -> [w322] mode=indexing
          n283 = call "SubVI Set Front panel elements.vi"("Enable elements (T)"=w323, "error in (passthrough)"=w326, "Array"=w327) -> ("error out"=w325:errorcluster)  [unwired: 8 in]
          n284 = call "SubVI Set Front panel elements.vi"("Enable elements (T)"=w323, "error in (passthrough)"=w325, "Array"=w322) -> ("error out"=w324:errorcluster)  [unwired: 8 in]
        }
        n285 = for {
          N: 2 -> [_]
          shift-right: [w331] -> w306
          shift-left: w311 -> [w330]
          i -> [w329]
          n286 = Increment(x=w329) -> (x+1=w328:i32)
          n287 = for {
            N: 6 -> [_]
            shift-right: [w340] -> w331
            shift-left: w330 -> [w339]
            tunnel: w328 -> [w334]
            i -> [w337]
            # "#XXX no way how to check guard status?"
            n288 = local read "VISA"() -> (w338:refnum<visa-resource-name>)
            n289 = Increment(x=w337) -> (x+1=w335:i32)
            n290 = call "Get Channel Status.vi"("Channel"=w334, "Slave"=w335, "error in (no error)"=w339, "VISA resource name"=w338) -> ("error out"=w340:errorcluster, "Channel Enabled"=w333:bool)  [unwired: 5 in, 1 out]
            n291 = local read "Slaves ref array"() -> (w336:refnum<vi>[][])
            n292 = call "SubVI Set FP Channel-Guard value.vi"("Value"=w333, "Ch ID"=w334, "Slave ID"=w335, "Slaves ref array"=w336) -> ()  [unwired: 7 in, 1 out]
          }
        }
        n293 = Enqueue Element(queue=w307, element="slaves update", error in (no error)=w306) -> (error out=w305:errorcluster)  [unwired: 1 in, 2 out]
        n294 = local read "FP"() -> (w320:refnum<vi>[])
        n295 = call "SubVI Set Front panel elements.vi"("error in (passthrough)"=w305, "Array"=w320) -> ("error out"=w321:errorcluster)  [unwired: 9 in]
        n296 = local write "error"(w321) -> ()
      }
      event "Get Status": Value Change {
        n297 = event-data() -> ()  [unwired: 1 in, 6 out]
        n298 = local read "FP"() -> (w359:refnum<vi>[])
        n299 = call "SubVI Set Front panel elements.vi"("Enable elements (T)"=FALSE, "Array"=w359) -> ("error out"=w354:errorcluster)  [unwired: 9 in]
        n300 = local read "VISA"() -> (w355:refnum<visa-resource-name>)
        n301 = call "Get MX Status.vi"("error in (no error)"=w354, "VISA resource name"=w355) -> ("error out"=w353:errorcluster, "Ready?"=→"Ready?":bool, "Enabled"=→"Enabled":bool, "TRG Polarity Positive"=w348:bool, "Local?"=w352:bool, "TRG External"=w344:bool)  [unwired: 3 in, 1 out]
        n302 = local read "FP"() -> (w360:refnum<vi>[])
        n303 = Select(t=enum32{"Remote", "Local"}."Local" ("Operation"), s=w352, f=enum32{"Remote", "Local"}."Remote" ("Operation")) -> (s? t:f=w349:enum32{"Remote", "Local"})
        n304 = Select(t=enum32{"Positive", "Negative"}."Positive" ("Trigger polarity"), s=w348, f=enum32{"Positive", "Negative"}."Negative" ("Trigger polarity")) -> (s? t:f=w345:enum32{"Positive", "Negative"})
        n305 = Select(t=enum32{"Internal", "External"}."External" ("Trigger source"), s=w344, f=enum32{"Internal", "External"}."Internal" ("Trigger source")) -> (s? t:f=w341:enum32{"Internal", "External"})
        n306 = call "SubVI Set Front panel elements.vi"("error in (passthrough)"=w353, "Array"=w360) -> ("error out"=w361:errorcluster)  [unwired: 9 in]
        n307 = local write "Operation"(w349) -> ()
        n308 = local write "Trigger polarity"(w345) -> ()
        n309 = local write "Trigger source"(w341) -> ()
        n310 = local write "error"(w361) -> ()
      }
      event "no sequences get": Value Change {
        n311 = event-data() -> ()  [unwired: 1 in, 6 out]
        n312 = local read "FP"() -> (w367:refnum<vi>[])
        n313 = call "SubVI Set Front panel elements.vi"("Enable elements (T)"=FALSE, "Array"=w367) -> ("error out"=w365:errorcluster)  [unwired: 9 in]
        n314 = local read "VISA"() -> (w363:refnum<visa-resource-name>)
        n315 = call "Get Number of Sequences.vi"("error in (no error)"=w365, "VISA resource name"=w363) -> ("error out"=w364:errorcluster, "Number of sequences"=w362:i32)  [unwired: 7 in, 1 out]
        n316 = local read "FP"() -> (w368:refnum<vi>[])
        n317 = local write "Number of sequence lines:"(w362) -> ()
        n318 = call "SubVI Set Front panel elements.vi"("error in (passthrough)"=w364, "Array"=w368) -> ("error out"=w369:errorcluster)  [unwired: 9 in]
        n319 = local write "error"(w369) -> ()
      }
      event "sequence editor": Value Change {
        n320 = event-data() -> ()  [unwired: 1 in, 6 out]
        n321 = Enqueue Element(queue=w371, element="FP open") -> ()  [unwired: 2 in, 3 out]
      }
      event "Load sq to MX": Value Change {
        n322 = event-data() -> ()  [unwired: 1 in, 6 out]
        n323 = disable-structure shown="Default" {
          disable-tunnel: w376 -> [w408]
          disable-tunnel: [w393] -> w375
          disable-tunnel: [w392] -> w374
          frame Enabled {
            # "Get actual values from Sequence editor.vi"
            n324 = property class="VI"(reference=w408) -> ("Panel"=w407:refnum<vi>)  [unwired: 1 in, 2 out]
            n325 = property class="Pnl"(reference=w407) -> (reference out=w394:refnum<vi>, "Controls[]"=w395:refnum<vi>[])  [unwired: 1 in, 1 out]
            n326 = Close Reference(reference=w394) -> ()  [unwired: 1 in, 1 out]
            n327 = Close Reference(reference=w395) -> ()  [unwired: 1 in, 1 out]
            n328 = for {
              tunnel: w395 -> [w410] mode=indexing
              tunnel: [w409] -> w397 mode=indexing
              n329 = property class="Ctl"(reference=w410) -> ("Label.Text"=w409:string)  [unwired: 1 in, 2 out]
            }
            n330 = call "Search Unsorted 1D Array.vim"("element"="Sequence" ("Label.Text"), "unsorted 1D array"=w397) -> ("index of element"=w399:i32)  [unwired: 9 in]
            n331 = call "Search Unsorted 1D Array.vim"("element"="Timing\ndelay" ("Label.Text"), "unsorted 1D array"=w397) -> ("index of element"=w405:i32)  [unwired: 9 in]
            n332 = Index Array(array=w395, index=w399) -> (element=w400:refnum<vi>)
            n333 = property class="Ctl"(reference=w400) -> ("Value"=w401:variant)  [unwired: 1 in, 2 out]
            n334 = Index Array(array=w395, index=w405) -> (element=w404:refnum<vi>)
            n335 = property class="Ctl"(reference=w404) -> ("Value"=w403:variant)  [unwired: 1 in, 2 out]
            n336 = Variant To Data(type=u8[] [] ("Ch. bytes 2"), Variant=w403) -> (data=w392:u8[])  [unwired: 1 in, 1 out]
            n337 = Variant To Data(type=bool[][] [], Variant=w401) -> (data=w393:bool[][])  [unwired: 1 in, 1 out]
          }
        }
        n338 = Array Size(array=w374) -> (size(s)=w373:i32)
        n339 = Equal To 0?(x=w373) -> (x = 0?=w372:bool)
        n340 = case shown="False" w372 {
          tunnel: w375 -> [w382 _]
          tunnel: w374 -> [w381 _]
          frame False {
            n341 = local read "FP"() -> (w386:refnum<vi>[])
            n342 = call "Sequences to Bytes.vi"("Channel states"=w382) -> ("Ch. bytes 2"=w389:u8[], "Ch. bytes 1"=w390:u8[])  [unwired: 9 in]
            n343 = call "SubVI Set Front panel elements.vi"("Enable elements (T)"=FALSE, "Array"=w386) -> ("error out"=w384:errorcluster)  [unwired: 9 in]
            n344 = local read "VISA"() -> (w383:refnum<visa-resource-name>)
            n345 = call "Load Sequences.vi"("Byte 2 Ch."=w389, "Byte 3 Timing Delay"=w381, "Byte 1 Ch."=w390, "error in (no error)"=w384, "VISA resource name"=w383) -> ("error out"=w379:errorcluster, "VISA resource name out"=w377:refnum<visa-resource-name>)  [unwired: 5 in]
            n346 = local read "FP"() -> (w387:refnum<vi>[])
            n347 = call "Get Number of Sequences.vi"("error in (no error)"=w379, "VISA resource name"=w377) -> ("error out"=w378:errorcluster, "Number of sequences"=w380:i32)  [unwired: 7 in, 1 out]
            n348 = call "SubVI Set Front panel elements.vi"("error in (passthrough)"=w378, "Array"=w387) -> ("error out"=w388:errorcluster)  [unwired: 9 in]
            n349 = local write "error"(w388) -> ()
            n350 = local write "Number of sequence lines:"(w380) -> ()
          }
          frame True {
            n351 = One Button Dialog(message="Sequence matrix is empty.\nUse sequence editor to create\nsequence or load sequence\nfrom file.") -> ()  [unwired: 1 in, 1 out]
          }
        }
      }
      event "set sq line": Value Change {
        n352 = event-data() -> ()  [unwired: 1 in, 6 out]
        n353 = disable-structure shown="Default" {
          disable-tunnel: w424 -> [w435]
          disable-tunnel: [w425] -> w419
          frame Enabled {
            # "Get actual values from Sequence editor.vi"
            n354 = property class="VI"(reference=w435) -> ("Panel"=w434:refnum<vi>)  [unwired: 1 in, 2 out]
            n355 = property class="Pnl"(reference=w434) -> (reference out=w426:refnum<vi>, "Controls[]"=w427:refnum<vi>[])  [unwired: 1 in, 1 out]
            n356 = Close Reference(reference=w426) -> ()  [unwired: 1 in, 1 out]
            n357 = Close Reference(reference=w427) -> ()  [unwired: 1 in, 1 out]
            n358 = for {
              tunnel: w427 -> [w437] mode=indexing
              tunnel: [w436] -> w429 mode=indexing
              n359 = property class="Ctl"(reference=w437) -> ("Label.Text"=w436:string)  [unwired: 1 in, 2 out]
            }
            n360 = call "Search Unsorted 1D Array.vim"("element"="Sequence" ("Label.Text"), "unsorted 1D array"=w429) -> ("index of element"=w431:i32)  [unwired: 9 in]
            n361 = Index Array(array=w427, index=w431) -> (element=w432:refnum<vi>)
            n362 = property class="Ctl"(reference=w432) -> ("Value"=w433:variant)  [unwired: 1 in, 2 out]
            n363 = Variant To Data(type=bool[][] [], Variant=w433) -> (data=w425:bool[][])  [unwired: 1 in, 1 out]
          }
        }
        n364 = Decrement(x="Set to sequence line:") -> (x-1=w411:i32)
        n365 = local read "FP"() -> (w422:refnum<vi>[])
        n366 = Index Array(array=w419, index (row)=w411) -> (element=w418:bool[])  [unwired: 1 in]
        n367 = call "SubVI Set Front panel elements.vi"("Enable elements (T)"=FALSE, "Array"=w422) -> ("error out"=w420:errorcluster)  [unwired: 9 in]
        n368 = local read "VISA"() -> (w417:refnum<visa-resource-name>)
        n369 = call "Set Sequence Line.vi"("error in (no error)"=w420, "Sequence Line"=w418, "VISA resource name"=w417) -> ("error out"=w416:errorcluster)  [unwired: 7 in, 1 out]
        n370 = local read "FP"() -> (w423:refnum<vi>[])
        n371 = call "SubVI Set Front panel elements.vi"("error in (passthrough)"=w416, "Array"=w423) -> ("error out"=w415:errorcluster)  [unwired: 9 in]
        n372 = property on="dummy for event \"check channels\"" class="Bool (strict)"(error in=w415, "Val(Sgnl)"=TRUE) -> (error out=w414:errorcluster)  [unwired: 1 in, 1 out]
        n373 = local write "error"(w414) -> ()
      }
      event "Get sq from MX": Value Change {
        n374 = event-data() -> ()  [unwired: 1 in, 6 out]
        n375 = local read "FP"() -> (w439:refnum<vi>[])
        n376 = call "SubVI Set Front panel elements.vi"("Enable elements (T)"=FALSE, "Array"=w439) -> ("error out"=w457:errorcluster)  [unwired: 9 in]
        n377 = local read "VISA"() -> (w455:refnum<visa-resource-name>)
        n378 = call "Get Sequences.vi"("error in (no error)"=w457, "VISA resource name"=w455) -> ("error out"=w456:errorcluster, "Byte 3 Delay"=w449:u8[], "Byte 2 Ch."=w452:u8[], "Byte 1 Ch."=w453:u8[])  [unwired: 5 in, 1 out]
        n379 = Array Size(array=w449) -> (size(s)=w454:i32)
        n380 = local read "FP"() -> (w458:refnum<vi>[])
        n381 = call "Bytes to Sequences.vi"("Ch. bytes 2"=w452, "Ch. bytes 1"=w453) -> ("Array"=w450:bool[][])  [unwired: 9 in]
        n382 = call "SubVI Set Front panel elements.vi"("error in (passthrough)"=w456, "Array"=w458) -> ("error out"=w459:errorcluster)  [unwired: 9 in]
        n383 = local write "Number of sequence lines:"(w454) -> ()
        n384 = local write "error"(w459) -> ()
        n385 = disable-structure shown="Default" {
          disable-tunnel: w451 -> [w473]
          disable-tunnel: w450 -> [w462]
          disable-tunnel: w449 -> [w461]
          disable-tunnel: w448 -> [w460]
          disable-tunnel: [w460] -> w440
          frame Enabled {
            # "Push actual values to Sequence editor.vi"
            n386 = property class="VI"(reference=w473) -> ("Panel"=w472:refnum<vi>)  [unwired: 1 in, 2 out]
            n387 = property class="Pnl"(reference=w472) -> (reference out=w463:refnum<vi>, "Controls[]"=w464:refnum<vi>[])  [unwired: 1 in, 1 out]
            n388 = Close Reference(reference=w463) -> ()  [unwired: 1 in, 1 out]
            n389 = Close Reference(reference=w464) -> ()  [unwired: 1 in, 1 out]
            n390 = for {
              tunnel: w464 -> [w475] mode=indexing
              tunnel: [w474] -> w465 mode=indexing
              n391 = property class="Ctl"(reference=w475) -> ("Label.Text"=w474:string)  [unwired: 1 in, 2 out]
            }
            n392 = call "Search Unsorted 1D Array.vim"("element"="Sequence" ("Label.Text"), "unsorted 1D array"=w465) -> ("index of element"=w467:i32)  [unwired: 9 in]
            n393 = call "Search Unsorted 1D Array.vim"("element"="Timing\ndelay" ("Label.Text"), "unsorted 1D array"=w465) -> ("index of element"=w470:i32)  [unwired: 9 in]
            n394 = Index Array(array=w464, index=w467) -> (element=w468:refnum<vi>)
            n395 = property class="Ctl"(reference=w468, "Value"=w462) -> ()  [unwired: 1 in, 2 out]
            n396 = Index Array(array=w464, index=w470) -> (element=w469:refnum<vi>)
            n397 = property class="Ctl"(reference=w469, "Value"=w461) -> ()  [unwired: 1 in, 2 out]
          }
        }
        n398 = Enqueue Element(queue=w440, element="sequence fill missing collumns") -> (queue out=w444:refnum<queue>, error out=w447:errorcluster)  [unwired: 2 in, 1 out]
        n399 = Enqueue Element(queue=w444, element="index timing update", error in (no error)=w447) -> (queue out=w445:refnum<queue>, error out=w446:errorcluster)  [unwired: 1 in, 1 out]
        n400 = Enqueue Element(queue=w445, element="scrollbar sync", error in (no error)=w446) -> ()  [unwired: 1 in, 3 out]
      }
    }
  }
  n401 = flat-sequence {
    tunnel: w9 -> [w479]
    tunnel: w10 -> [w476]
    tunnel: w13 -> [_]
    tunnel: [w479] -> w3
    tunnel: [w477] -> w1
    tunnel: [w486] -> w5
    tunnel: ["Do full quit? (T)"] -> w4
    tunnel: w3 -> [w486]
    tunnel: [w480] -> w2
    tunnel: w1 -> [w480]
    tunnel: w4 -> [w491]
    tunnel: w5 -> [w490]
    tunnel: w2 -> [w488]
    frame #0 {
      n402 = Enqueue Element(queue=w476, element="quit") -> (error out=w477:errorcluster)  [unwired: 2 in, 2 out]
    }
    frame #1 {
      n403 = property class="VI"() -> ("FP.State"=w485:T2)  [unwired: 2 in, 2 out]
      n404 = Not Equal?(x=w485, y=T2."Closed") -> (x != y?=w482:bool)
      n405 = Compound Arithmetic op=AND(invert "Do full quit? (T)", w482) -> (w481:bool)
      n406 = case shown="True" w481 {
        tunnel: w486 -> [_ w487]
        frame False {
        }
        frame True {
          n407 = invoke class="VI" method="FP.Close"(reference=w487) -> ()  [unwired: 2 in, 3 out]
        }
      }
    }
    frame #2 {
      n408 = local read "VISA"() -> (w494:refnum<visa-resource-name>)
      n409 = call "Close.vi"("VISA resource name"=w494) -> ("error out"=w493:errorcluster)  [unwired: 10 in]
      n410 = Close Reference(reference=w490) -> (error out=w489:errorcluster)  [unwired: 1 in]
      n411 = Merge Errors(w493, w488, w489) -> (w492:errorcluster)
      "error" <- w492
      n412 = case shown="True" w491 {
        tunnel: w492 -> [_ w495]
        frame False {
        }
        frame True {
          n413 = disable-structure shown="RUN_TIME_ENGINE==True" {
            disable-tunnel: w495 -> [_ _]
            frame condition #0 (active) {
              n414 = Stop(stop? (T)=TRUE) -> ()
            }
            frame condition #1 {
              n415 = Quit LabVIEW(quit? (T)=TRUE) -> ()
            }
          }
        }
      }
    }
  }
